vi "respCleaner.vi"(2 "Garbage Start(0)":i32, 3 "Garbage Length(3)":i32=3, 4 "Delimiter (\\n)":string="\n", 5 "Raw Response":string) -> (0 "Data+Garbage":string[](array[string]), 1 "Clean Data":string[](array[string]))   [LabVIEW 2019]
uses:
  071376f2-fb96-48e1-b895-8ff016446a6e.vi
panel:
  out "Array 2":i32[](array[numeric])
  out "Array":bool[](array[boolean])
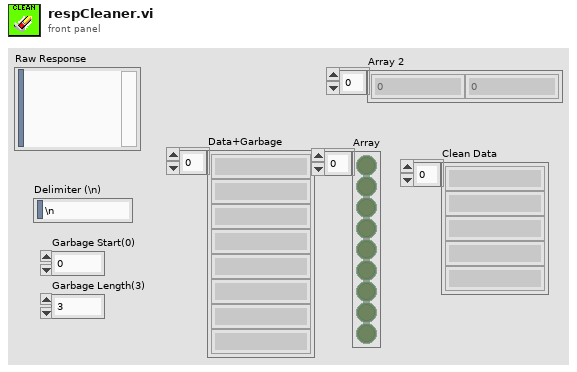
[diagram p1: front panel]
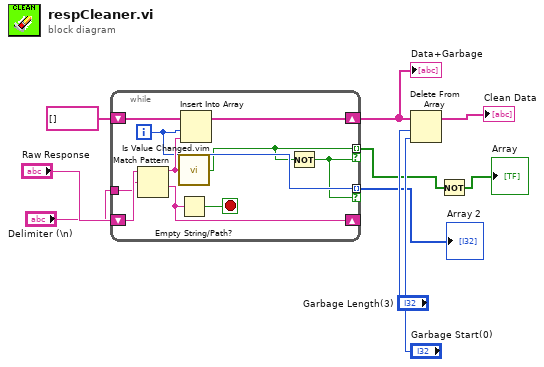
[diagram p0: block diagram]
diagram:
  n1 = while {
    tunnel: "Delimiter (\\n)" -> [w19]
    shift-right: [w16] -> _
    shift-left: "Raw Response" -> [w20]
    shift-right: [w17] -> w1
    shift-left: string[] [] -> [w18]
    tunnel: [w12] -> w4 mode=indexing if=w11
    tunnel: [w13] -> w2 mode=indexing if=w11
    i -> [w13]
    stop <- w15 stop-if-true
    n2 = Match Pattern(string=w20, regular expression=w19) -> (before substring=w14:string, after substring=w16:string)  [unwired: 1 in, 2 out]
    n3 = call "Is Value Changed.vim"("value"=w14) -> ("changed or first call?"=w12:bool)
    n4 = Empty String/Path?(string/path=w16) -> (empty?=w15:bool)
    n5 = Insert Into Array(array=w18, index=w13, new element=w14) -> (w17:string[])
    n6 = Not(x=w12) -> (.not. x?=w11:bool)
  }
  "Data+Garbage" <- w1
  "Array 2" <- w2
  n7 = Delete From Array(array=w1, length="Garbage Length(3)", index="Garbage Start(0)") -> (array with subset deleted=→"Clean Data":string[])  [unwired: 1 out]
  n8 = Not(x=w4) -> (.not. x?=→"Array":bool[])
